vi "number in array (SubVI).vi"(10 "Numeric":i32, 11 "Array":i32[](array[numeric])) -> (2 "indexes":i32[](array[numeric]), 3 "number":i32)   [LabVIEW 2020]
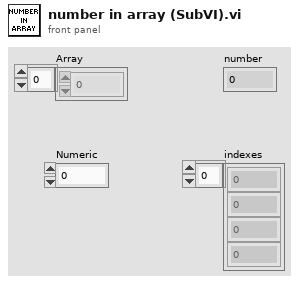
[diagram p1: front panel]
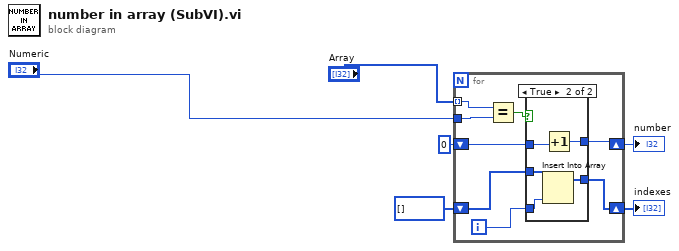
[diagram p0: block diagram]
diagram:
  n1 = for {
    tunnel: "Array" -> [w14] mode=indexing
    tunnel: "Numeric" -> [w13]
    shift-right: [w11] -> w6
    shift-left: 0 -> [w10]
    shift-right: [w8] -> w5
    shift-left: i32[] [] -> [w7]
    i -> [w9]
    n2 = Equal?(x=w14, y=w13) -> (x = y?=w12:bool)
    n3 = case shown="True" w12 {
      tunnel: [w16 w21] -> w11
      tunnel: w10 -> [w16 w20]
      tunnel: w9 -> [_ w18]
      tunnel: [w15 w19] -> w8
      tunnel: w7 -> [w15 w17]
      frame False {
      }
      frame True {
        n4 = Insert Into Array(array=w17, new element=w18) -> (w19:i32[])  [unwired: 1 in]
        n5 = Increment(x=w20) -> (x+1=w21:i32)
      }
    }
  }
  "indexes" <- w5
  "number" <- w6
